vi "MaynuoM9714.vi"(4 "error in":T13, 7 "Command":T14) -> (0 "error out":T13, 3 "Response":T11)   [LabVIEW 2018]
uses:
  MOKO_LabViewLibrary/MokoLowLevel/MokoLowLovelControl/MLLC_Command.ctl
  MOKO_LabViewLibrary/MokoLowLevel/MokoLowLovelControl/MLLC_Error.ctl
  MOKO_LabViewLibrary/MokoLowLevel/MokoLowLovelControl/MLLC_Mode.ctl
  MOKO_LabViewLibrary/MokoLowLevel/MokoLowLovelControl/MLLC_Response.ctl
  MOKO_LabViewLibrary/MokoLowLevel/MokoLowLovelControl/MLLC_DriverName.ctl
  MOKO_LabViewLibrary/MokoLowLevel/MokoLowLovelControl/MLLC_Request.ctl
  MOKO_LabViewLibrary/MokoLowLevel/MokoLowLovelControl/MLLC_ErrorCode.ctl
  MOKO_LabViewLibrary/MokoLowLevel/MokoLowLovelControl/MLLC_ResponseInit.ctl
  MOKO_LabViewLibrary/MokoLowLevel/MokoLowLovelControl/MLLC_ConnectCluster.ctl
  MOKO_LabViewLibrary/MokoLowLevel/MokoLowLovelControl/MLLC_InterfaceType.ctl
  MOKO_LabViewLibrary/MokoLowLevel/MokoLowLovelControl/MLLC_OpenedSession.ctl
  MOKO_LabViewLibrary/MokoLowLevel/MokoLowLovelControl/MLLC_InterfaceSettings.ctl
  MOKO_LabViewLibrary/MokoLowLevel/MokoLowLovelControl/MLLC_InterfaceKind.ctl
  MOKO_LabViewLibrary/MokoLowLevel/MokoLowLovelControl/MLLC_Rs232Settings.ctl
  data/M97-98 Series DC Electronic Load LabVIEW Driver/M9700 Driver/86/vi.lib/M9700 Modbus.llb/CTL Register Address.ctl
  data/M97-98 Series DC Electronic Load LabVIEW Driver/M9700 Driver/86/vi.lib/M9700 Modbus.llb/CTL CMD Register.ctl
panel:
  in  "Settings":T6={"Saved Data"=variant, "Data"={"Connect"={"InterfaceType"=enum."VISA", "OpenedSession"="", "InterfaceSettings"={"Interface"=enum."GPIB", "EOS 4 read"=enum."LF (\\n)", "EOS 4 write"=enum."LF (\\n)", "TMO, ms"=5000, "Sett"=variant(cluster{"Baud Rate":u32, "Data Bits":u16, "Parity":u16, "Stop Bits":u16, "Flow Control":u16, "Eho":bool} {"Baud Rate"=75, "Data Bits"=0, "Parity"=0, "Stop Bits"=0, "Flow Control"=0, "Eho"=FALSE})}}}}
  in  "Response Init":T7
  in  "Error Code":T8=5475
  in  "Request":T9
  in  "Driver Name":T10="MaynuoM9714"
  in  "Mode":T12=enum."Check"
  # "MaynuoM9714"
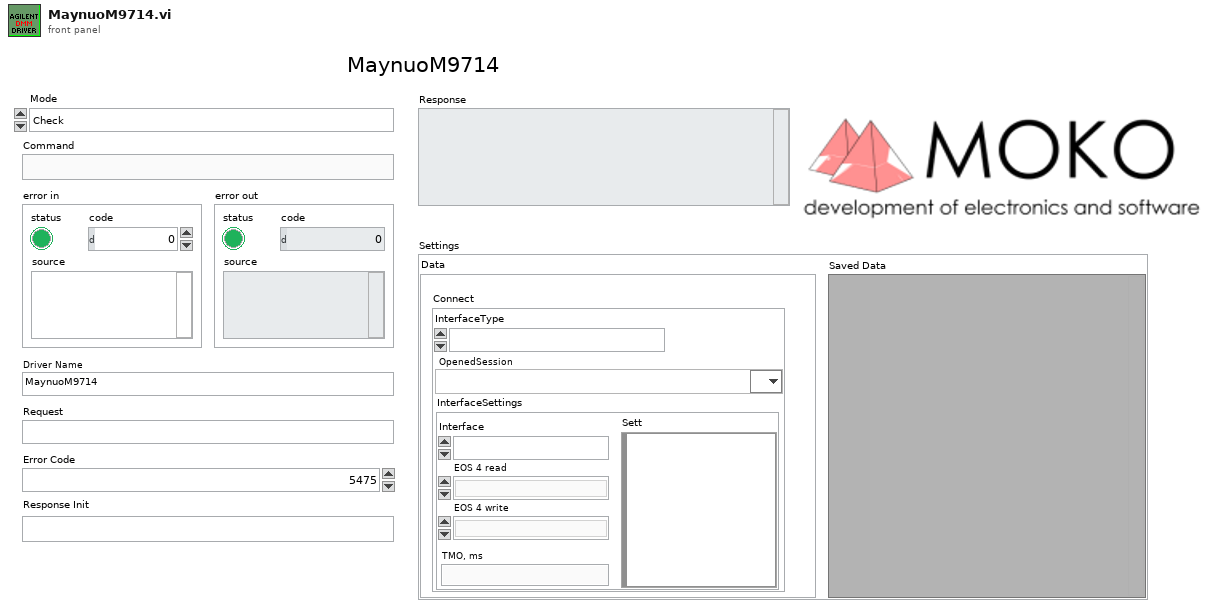
[diagram p1: front panel]
types:
  T1 = typedef "MLLC_ConnectCluster.ctl" = cluster{"InterfaceType":T2, "OpenedSession":T3, "InterfaceSettings":T4}
  T2 = typedef "MLLC_InterfaceType.ctl" = enum16{"VISA", "Prologix USB-GPIB"}
  T3 = typedef "MLLC_OpenedSession.ctl" = refnum<visa-resource-name>
  T4 = typedef "MLLC_InterfaceSettings.ctl" = cluster{"Interface":T5, "EOS 4 read":enum16{"Default (=EOS 4 write)", "CR (\\r)", "LF (\\n)", "None"}, "EOS 4 write":enum16{"CR+LF (\\r\\n)", "CR (\\r)", "LF (\\n)", "None"}, "TMO, ms":i32, "Sett":variant}
  T5 = typedef "MLLC_InterfaceKind.ctl" = enum16{"RS232", "GPIB", "USB", "Ethernet", "another"}
  T6 = cluster{"Saved Data":variant, "Data":cluster{"Connect":T1}}
  T7 = typedef "MLLC_ResponseInit.ctl" = string
  T8 = typedef "MLLC_ErrorCode.ctl" = u32
  T9 = typedef "MLLC_Request.ctl" = string
  T10 = typedef "MLLC_DriverName.ctl" = string
  T11 = typedef "MLLC_Response.ctl" = string
  T12 = typedef "MLLC_Mode.ctl" = enum16{"get", "set", "close", "Init", "Check"}
  T13 = typedef "MLLC_Error.ctl" = errorcluster
  T14 = typedef "MLLC_Command.ctl" = string
  T15 = typedef "MLLC_Rs232Settings.ctl" = cluster{"Baud Rate":u32, "Data Bits":u16, "Parity":u16, "Stop Bits":u16, "Flow Control":u16, "Eho":bool, "Address":dbl}
  T16 = typedef "CTL CMD Register.ctl" = u8
  T17 = typedef "CTL Register Address.ctl" = u16
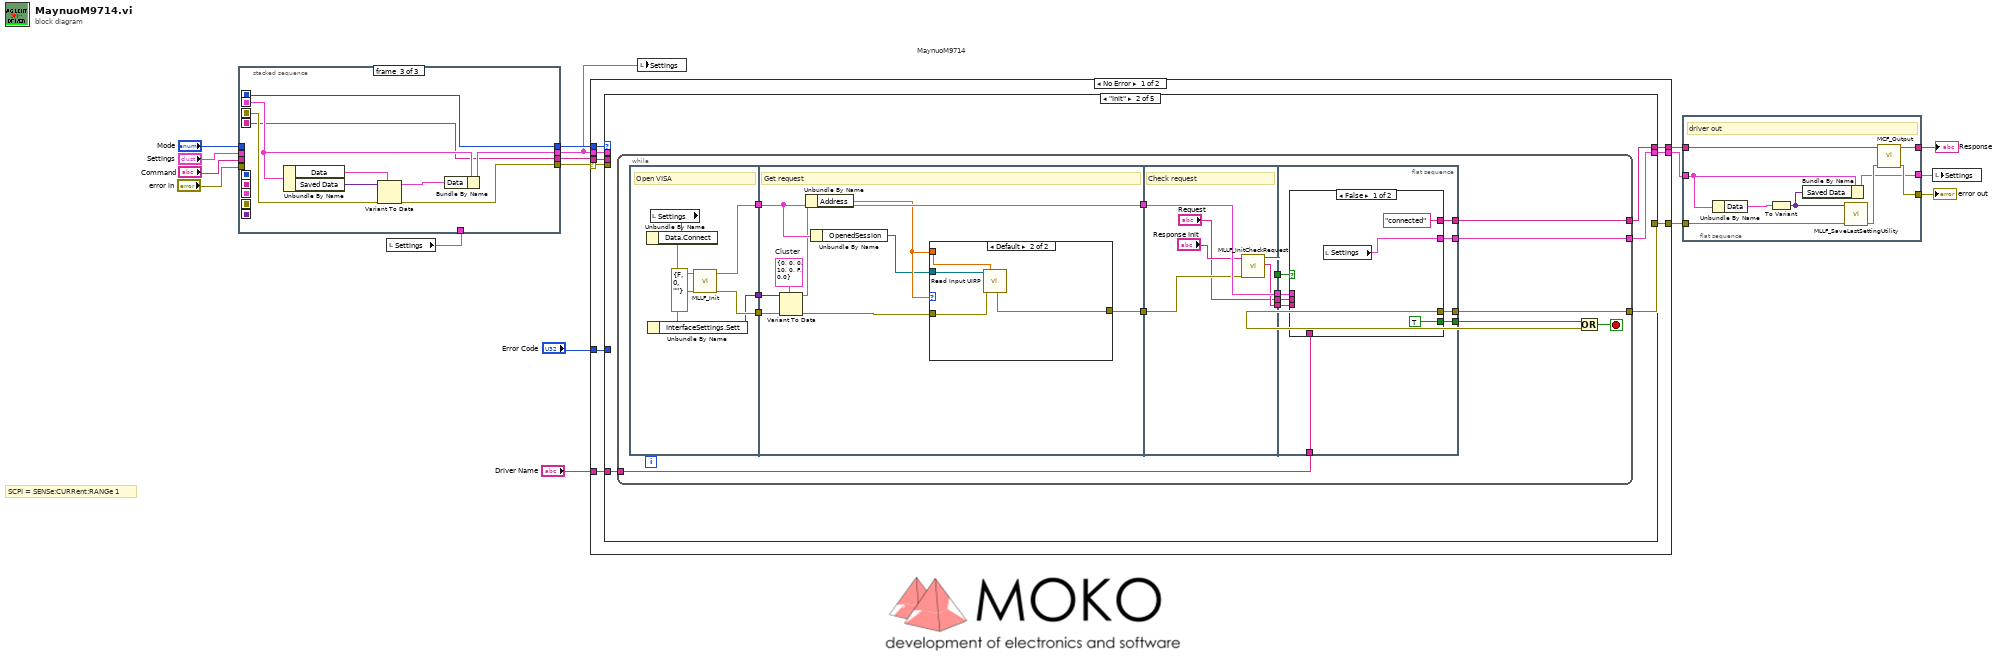
[diagram p0: block diagram]
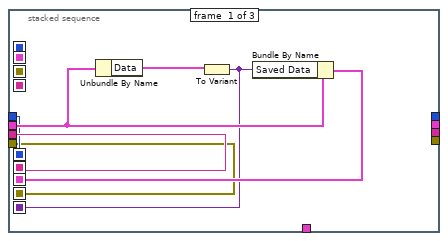
[diagram p2: hidden frame]
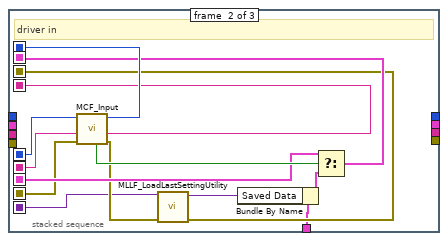
[diagram p3: hidden frame]
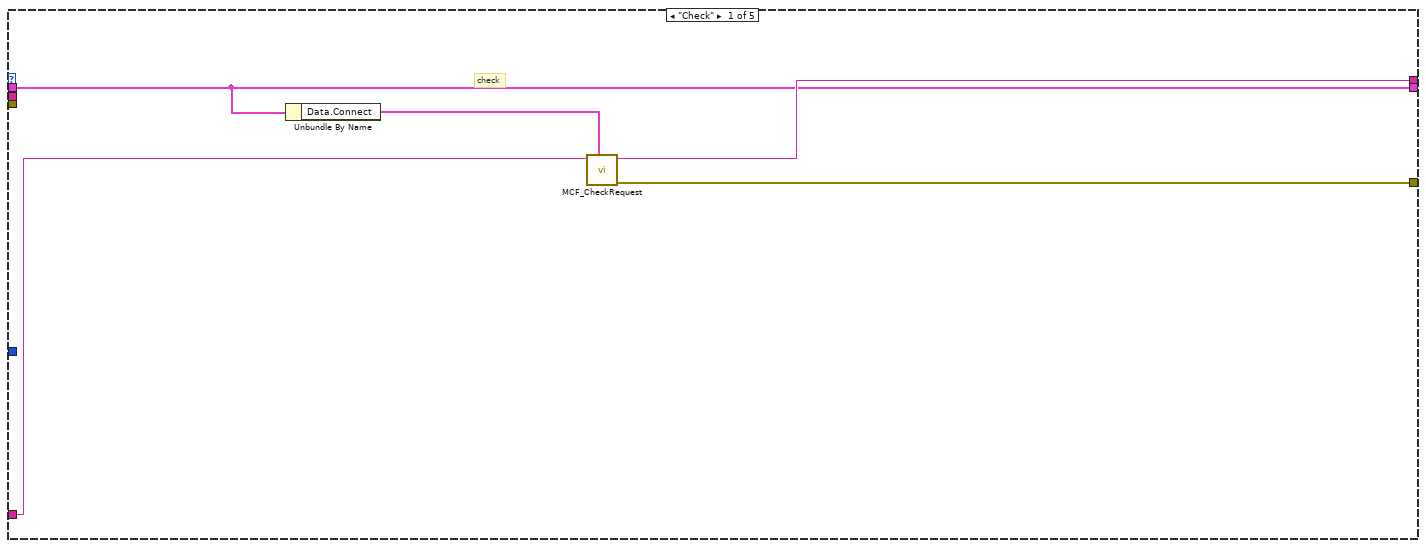
[diagram p4: hidden frame]
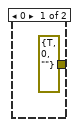
[diagram p5: hidden frame]
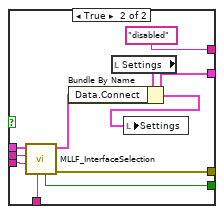
[diagram p6: hidden frame]
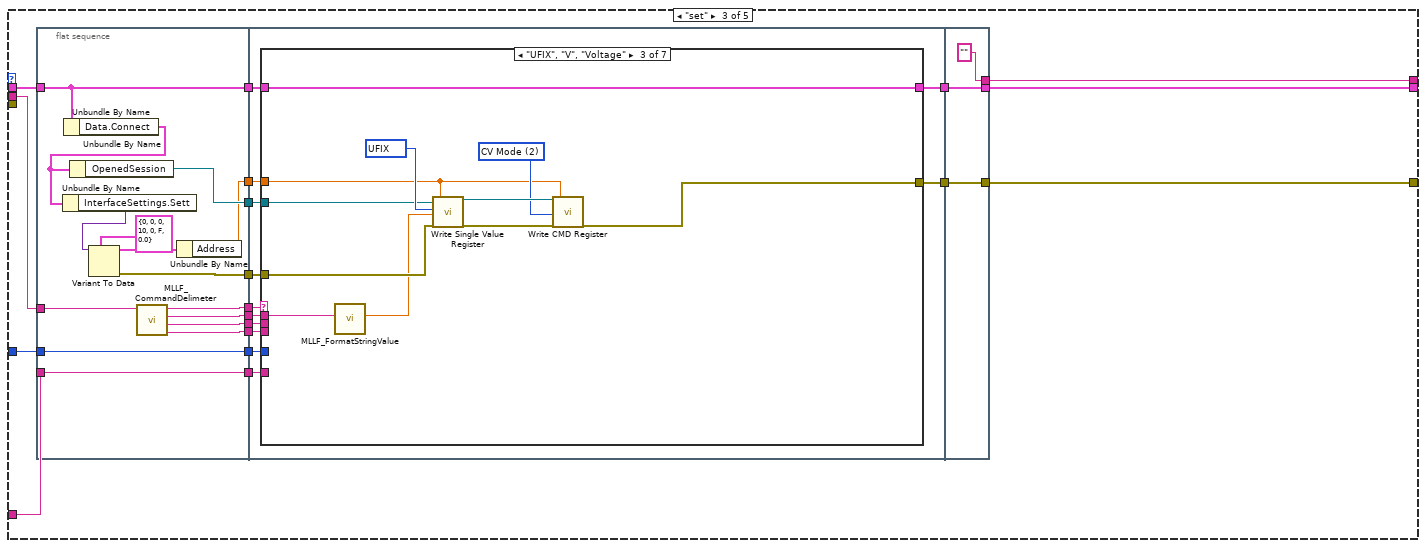
[diagram p7: hidden frame]
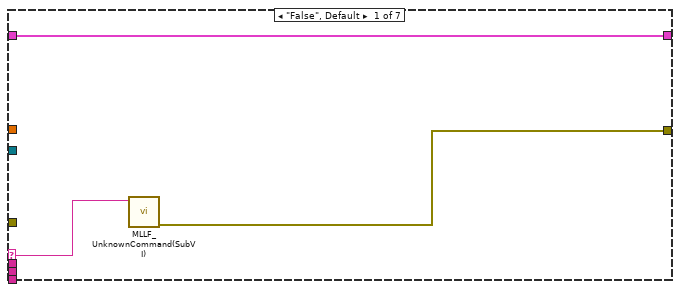
[diagram p8: hidden frame]
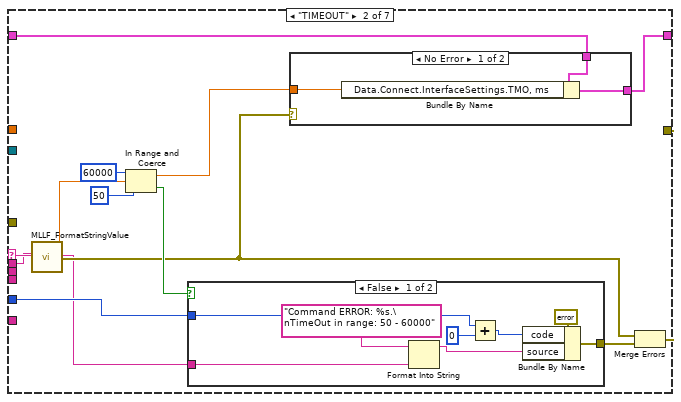
[diagram p9: hidden frame]
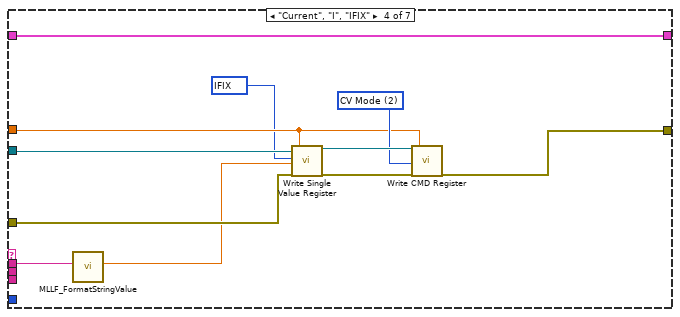
[diagram p12: hidden frame]
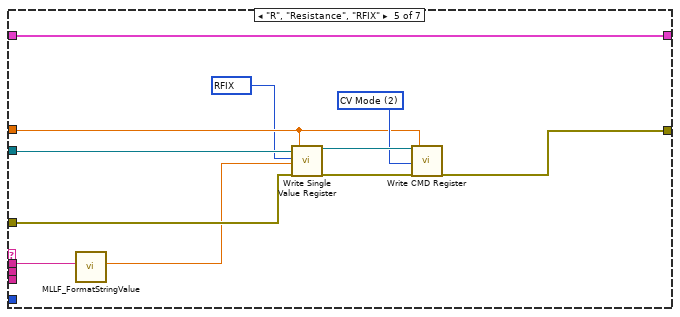
[diagram p13: hidden frame]
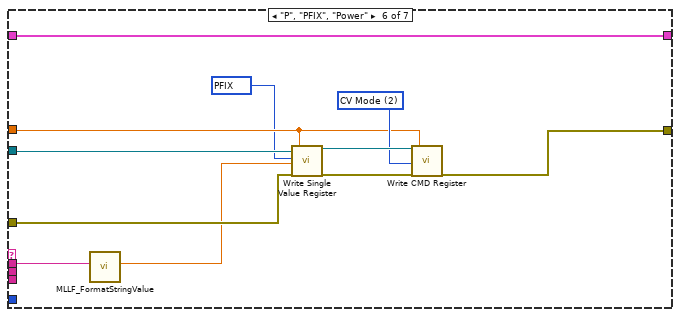
[diagram p14: hidden frame]
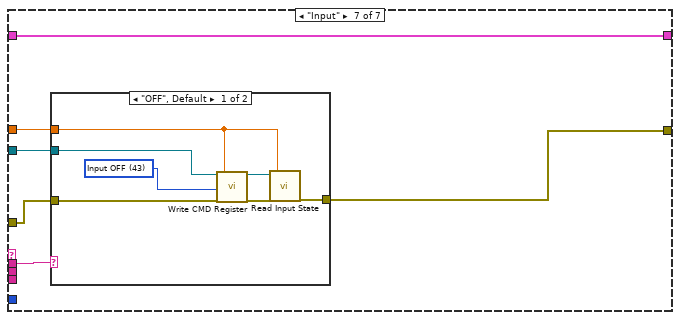
[diagram p15: hidden frame]
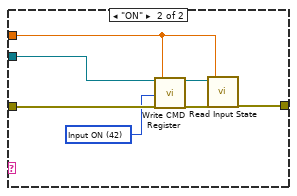
[diagram p16: hidden frame]
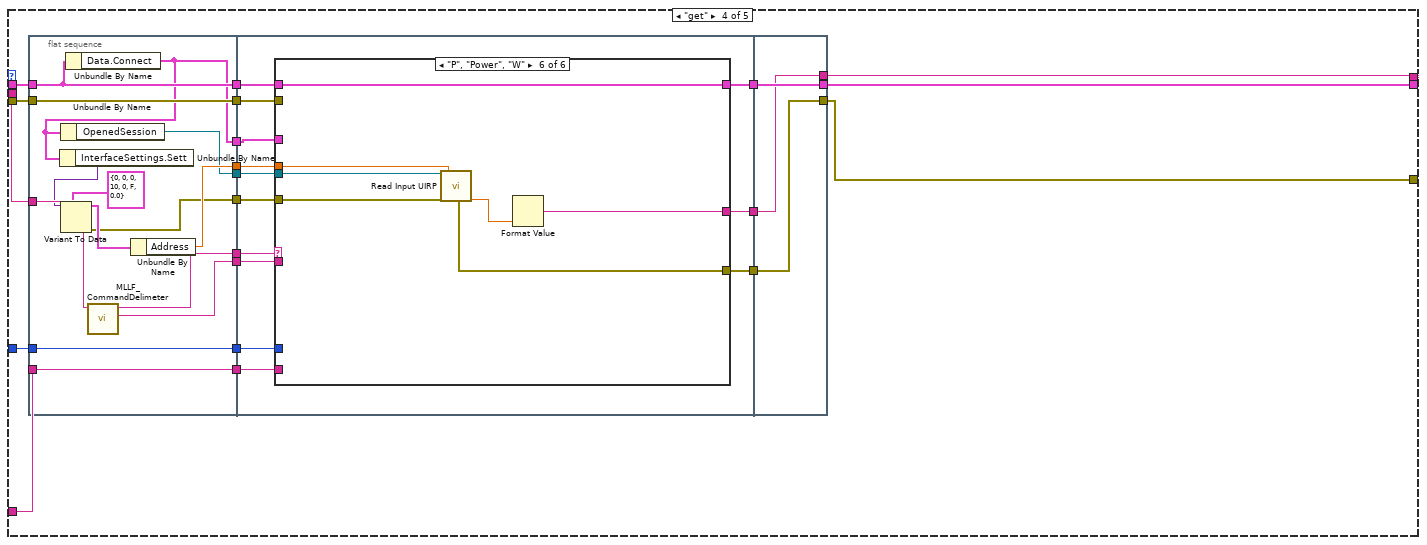
[diagram p17: hidden frame]
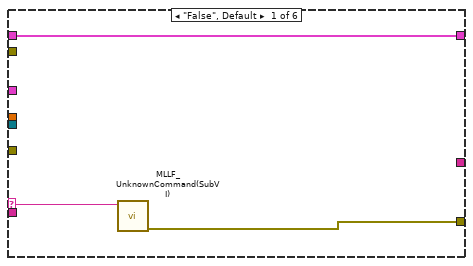
[diagram p18: hidden frame]
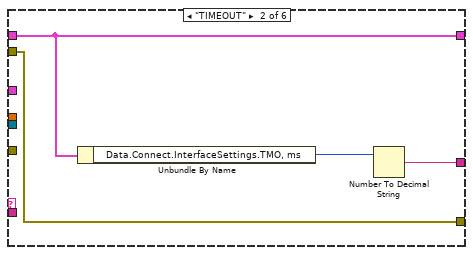
[diagram p19: hidden frame]
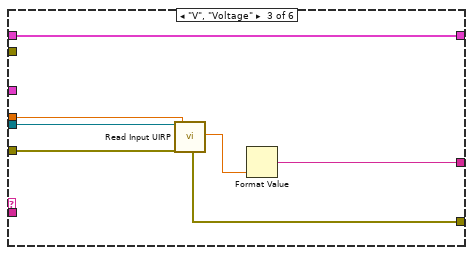
[diagram p20: hidden frame]
diagram:
  # "SCPI = SENSe:CURRent:RANGe 1"
  # "MaynuoM9714"
  n1 = local read "Settings"() -> (w8:T6)
  n2 = stacked-sequence {
    seq-local: [w20 _ _] -> [_ w36 _]
    seq-local: [w19 _ _] -> [_ w37 _]
    seq-local: [w22 _ _] -> [_ w32 _]
    seq-local: [w18 _ _] -> [_ w31 _]
    seq-local: [w21 _ _] -> [_ w27 _]
    seq-local: [_ w28 _] -> [_ _ w44]
    seq-local: [_ w38 _] -> [_ _ w41]
    seq-local: [_ w35 _] -> [_ _ w40]
    seq-local: [_ w34 _] -> [_ _ w45]
    tunnel: "Command" -> [w20 _ _]
    tunnel: "Mode" -> [w19 _ _]
    tunnel: "error in" -> [w18 _ _]
    tunnel: "Settings" -> [w23 _ _]
    tunnel: w8 -> [_ w26 _]
    tunnel: [_ _ w40] -> w10
    tunnel: [_ _ w43] -> w1
    tunnel: [_ _ w42] -> w9
    tunnel: [_ _ w41] -> w11
    frame #0 {
      n3 = Unbundle By Name(w23) -> ("Data"=w24:cluster{"Connect":T1})
      n4 = To Variant(anything=w24) -> (Variant=w21:variant)
      n5 = Bundle By Name(cluster=w23, "Saved Data"=w21) -> (w22:T6)
    }
    frame #1 {
      # "driver in"
      n6 = call "MCF_Input.vi"("Error In"=w31, "Command in"=w36, "Mode in"=w37) -> ("Error Out"=w30:errorcluster, "Command out"=w35:string, "Mode out"=w38:T12, "Boolean"=w33:bool)  [unwired: 5 in]
      n7 = call "MLLF_LoadLastSettingUtility.vi"("Error In"=w30, "Save data in"=w27) -> ("Error Out"=w28:errorcluster, "Save data out"=w25:variant)  [unwired: 8 in]
      n8 = Bundle By Name(cluster=w26, "Saved Data"=w25) -> (w29:T6)
      n9 = Select(t=w32, s=w33, f=w29) -> (s? t:f=w34:T6)
    }
    frame #2 {
      n10 = Unbundle By Name(w45) -> ("Data"=w46:cluster{"Connect":T1}, "Saved Data"=w39:variant)
      n11 = Variant To Data(error in=w44, type=w46, Variant=w39) -> (data=w47:cluster{"Connect":T1}, error out=w42:errorcluster)
      n12 = Bundle By Name(cluster=w45, "Data"=w47) -> (w43:T6)
    }
  }
  n13 = case shown="No Error" w9 {
    selector: w9 -> [w53 w362]
    tunnel: [w54 w362] -> w5
    tunnel: w11 -> [w56 _]
    tunnel: [w55 "An error occurred in the driver input module." ("String")] -> w7
    tunnel: w10 -> [w48 _]
    tunnel: w1 -> [w49 w361]
    tunnel: "Error Code" -> [w52 _]
    tunnel: "Driver Name" -> [w51 _]
    tunnel: [w50 w361] -> w6
    frame No Error {
      n14 = case shown="\"Init\"" w56 {
        tunnel: [w60 w65 w141 w273 "" ("String")] -> w55
        tunnel: [w61 w63 w144 w274 w358] -> w54
        tunnel: w53 -> [_ _ _ w287 _]
        tunnel: w52 -> [_ _ w147 w289 _]
        tunnel: w51 -> [w59 w62 w145 w288 _]
        tunnel: [w58 w64 w146 w290 w357] -> w50
        tunnel: w49 -> [w58 _ w133 w279 w357]
        tunnel: w48 -> [_ _ w132 w278 _]
        frame "Check" {
          # "check"
          n15 = Unbundle By Name(w58) -> ("Data.Connect"=w57:T1)
          n16 = call "MCF_CheckRequest.vi"("Permanent data.Connect"=w57, "Driver Name"=w59) -> ("Error Out"=w61:errorcluster, "Output String"=w60:string)  [unwired: 8 in]
        }
        frame "Init" {
          n17 = while {
            tunnel: [w71] -> w63
            tunnel: [w70] -> w65
            tunnel: [w69] -> w64
            tunnel: w62 -> [w73]
            stop <- w80 stop-if-true
            n18 = flat-sequence {
              tunnel: [w86] -> w79
              tunnel: [w85] -> w78
              tunnel: [w82] -> w66
              tunnel: w79 -> [w91]
              tunnel: w78 -> [w94]
              tunnel: [w95] -> w77
              tunnel: [w94] -> w76
              tunnel: w66 -> [w90]
              tunnel: w77 -> [w104]
              tunnel: w76 -> [w106]
              tunnel: [w106] -> w75
              tunnel: [w103] -> w74
              tunnel: [w102] -> w68
              tunnel: ["Request"] -> w67
              tunnel: w75 -> [w114]
              tunnel: w74 -> [w115]
              tunnel: w73 -> [w113]
              tunnel: [w112] -> w72
              tunnel: [w111] -> w71
              tunnel: [w110] -> w70
              tunnel: [w109] -> w69
              tunnel: w68 -> [w108]
              tunnel: w67 -> [w107]
              frame #0 {
                # "Open VISA"
                n19 = local read "Settings"() -> (w84:T6)
                n20 = Unbundle By Name(w84) -> ("Data.Connect"=w83:T1)
                n21 = Unbundle By Name(w83) -> ("InterfaceSettings.Sett"=w82:variant)
                n22 = call "MLLF_Init.vi"("Error In"=errorcluster {"status"=FALSE, "code"=0, "source"=""}, "DriverConnect in"=w83) -> ("Error Out"=w86:errorcluster, "DriverConnect out"=w85:T1)  [unwired: 6 in]
              }
              frame #1 {
                w92 = T15 {"Baud Rate"=0, "Data Bits"=0, "Parity"=0, "Stop Bits"=10, "Flow Control"=0, "Eho"=FALSE, "Address"=0.0}  # Cluster
                # "Get request"
                n23 = Variant To Data(error in=w91, type=w92, Variant=w90) -> (data=w93:T15, error out=w87:errorcluster)
                n24 = Unbundle By Name(w93) -> ("Address"=w89:dbl)
                n25 = Unbundle By Name(w94) -> ("OpenedSession"=w88:T3)
                n26 = case shown="Default" w89 {
                  tunnel: [errorcluster {"status"=TRUE, "code"=0, "source"=""} ("error out") w100] -> w95
                  tunnel: w88 -> [_ w99]
                  tunnel: w87 -> [_ w98]
                  tunnel: w89 -> [_ w97]
                  frame 0 {
                  }
                  frame Default {
                    n27 = call "Read Input UIRP.vi"("VISA resource name"=w99, "error in"=w98, "Load Address"=w97) -> ("error out"=w100:errorcluster)  [unwired: 16 out]
                  }
                }
              }
              frame #2 {
                # "Check request"
                n28 = call "MLLF_InitCheckRequest.vi"("error in (no error)"=w104, "Response Init"="Response Init") -> ("ResponseInit out"=w102:string, "Design"=w103:bool)  [unwired: 6 in, 2 out]
              }
              frame #3 {
                n29 = case shown="False" w115 {
                  tunnel: w114 -> [_ w127]
                  tunnel: [TRUE w122] -> w112
                  tunnel: [_ w125] -> w111
                  tunnel: ["connected" "disabled"] -> w110
                  tunnel: [w116 w123] -> w109
                  tunnel: w113 -> [_ w121]
                  tunnel: w108 -> [_ w120]
                  tunnel: w107 -> [_ w119]
                  frame False {
                    n30 = local read "Settings"() -> (w116:T6)
                  }
                  frame True {
                    n31 = call "MLLF_InterfaceSelection.vi"("Driver Name"=w121, "Response"=w120, "Request"=w119, "DriverConnect in"=w127) -> ("error out"=w125:T13, "DriverConnect out"=w126:T1, "stop init?"=w122:bool)  [unwired: 3 in, 2 out]
                    n32 = local read "Settings"() -> (w128:T6)
                    n33 = Bundle By Name(cluster=w128, "Data.Connect"=w126) -> (w123:T6)
                    n34 = local write "Settings"(w123) -> ()
                  }
                }
              }
            }
            n35 = Or(x=w72, y=w71) -> (x .or. y?=w80:bool)
          }
        }
        frame "set" {
          n36 = flat-sequence {
            tunnel: w145 -> [w161]
            tunnel: w133 -> [w155]
            tunnel: w147 -> [w162]
            tunnel: [w162] -> w140
            tunnel: [w155] -> w139
            tunnel: [w161] -> w138
            tunnel: [w156] -> w137
            tunnel: [w157] -> w136
            tunnel: [w158] -> w135
            tunnel: [w159] -> w134
            tunnel: w132 -> [w160]
            tunnel: [w152] -> w131
            tunnel: [w151] -> w130
            tunnel: [w150] -> w129
            tunnel: [w172] -> w143
            tunnel: [w168] -> w142
            tunnel: w140 -> [w174]
            tunnel: w139 -> [w173]
            tunnel: w138 -> [w171]
            tunnel: w137 -> [w170]
            tunnel: w136 -> [w169]
            tunnel: w135 -> [w167]
            tunnel: w134 -> [w166]
            tunnel: w131 -> [w165]
            tunnel: w130 -> [w164]
            tunnel: w129 -> [w163]
            tunnel: [w268] -> w144
            tunnel: [w269] -> w146
            tunnel: w143 -> [w269]
            tunnel: w142 -> [w268]
            tunnel: ["" ("String")] -> w141
            frame #0 {
              n37 = Unbundle By Name(w155) -> ("Data.Connect"=w149:T1)
              n38 = Unbundle By Name(w149) -> ("InterfaceSettings.Sett"=w148:variant)
              n39 = Unbundle By Name(w149) -> ("OpenedSession"=w152:T3)
              n40 = Variant To Data(type=T15 {"Baud Rate"=0, "Data Bits"=0, "Parity"=0, "Stop Bits"=10, "Flow Control"=0, "Eho"=FALSE, "Address"=0.0} ("Cluster"), Variant=w148) -> (data=w154:T15, error out=w150:errorcluster)  [unwired: 1 in]
              n41 = call "MLLF_CommandDelimeter.vi"("command with param"=w160) -> ("param 3"=w159:string, "param 2"=w158:string, "param 1"=w157:string, "command"=w156:string)  [unwired: 6 in, 1 out]
              n42 = Unbundle By Name(w154) -> ("Address"=w151:dbl)
            }
            frame #1 {
              n43 = case shown="\"UFIX\", \"V\", \"Voltage\"" w170 {
                selector: w170 -> [w176 w179 _ _ _ _ _]
                tunnel: w169 -> [_ w178 w204 w215 w226 w237 w247]
                tunnel: [w175 w184 w208 w220 w231 w242 w248] -> w168
                tunnel: w174 -> [_ w185 _ _ _ _ _]
                tunnel: w173 -> [w177 w189 w213 w224 w235 w246 w252]
                tunnel: [w177 w190 w213 w224 w235 w246 w252] -> w172
                tunnel: w171 -> [_ _ _ _ _ _ _]
                tunnel: w167 -> [_ _ _ _ _ _ _]
                tunnel: w166 -> [_ _ _ _ _ _ _]
                tunnel: w165 -> [_ _ w207 w219 w230 w241 w250]
                tunnel: w164 -> [_ _ w206 w218 w229 w240 w251]
                tunnel: w163 -> [_ _ w205 w217 w228 w239 w249]
                frame "False", Default {
                  n44 = call "MLLF_UnknownCommand(SubVI).vi"("Unknown command"=w176) -> ("error out"=w175:errorcluster)  [unwired: 10 in]
                }
                frame "TIMEOUT" {
                  n45 = call "MLLF_FormatStringValue.vi"("String Value"=w178) -> ("error out"=w180:T13, "number"=w181:dbl)  [unwired: 8 in, 1 out]
                  n46 = In Range and Coerce(upper limit=60000, x=w181, lower limit=50) -> (coerced(x)=w186:dbl, In Range?=w182:bool)
                  n47 = case shown="False" w182 {
                    tunnel: [w197 _] -> w183
                    tunnel: w185 -> [w196 _]
                    tunnel: w179 -> [w195 _]
                    frame False {
                      n48 = Format Into String(format string="Command ERROR: %s.\nTimeOut in range: 50 - 60000", w195) -> (resulting string=w199:string)  [unwired: 2 in, 1 out]
                      n49 = Add(x=w196, y=0) -> (x+y=w200:T8)
                      n50 = Bundle By Name(cluster=errorcluster {"status"=TRUE, "code"=0, "source"=""} ("error out"), "code"=w200, "source"=w199) -> (w197:errorcluster)
                    }
                    frame True {
                    }
                  }
                  n51 = case shown="No Error" w180 {
                    tunnel: [w193 w194] -> w190
                    tunnel: w189 -> [w192 w194]
                    tunnel: w186 -> [w191 _]
                    frame No Error {
                      n52 = Bundle By Name(cluster=w192, "Data.Connect.InterfaceSettings.TMO, ms"=w191) -> (w193:T6)
                    }
                    frame Error {
                    }
                  }
                  n53 = Merge Errors(w180, w183) -> (w184:errorcluster)
                }
                frame "UFIX", "V", "Voltage" {
                  w210 = T16 2 items=["CC Mode"=1, "CV Mode"=2, "CW Mode"=3, "CR Mode"=4, "Short Mode"=26, "Set SysPara"=41, "Input ON"=42, "Input OFF"=43] ("CMD Register Value")
                  w212 = T17 2563 items=["REMOTE"=1283, "ISTATE"=1296, "CMD"=2560, "IFIX"=2561, "UFIX"=2563, "PFIX"=2565, "RFIX"=2567, "IMAX"=2612, "UMAX"=2614, "PMAX"=2616, "U"=2816, "I"=2818, "MODEL"=2822, "EDITION"=2823] ("Register Address")
                  n54 = call "MLLF_FormatStringValue.vi"("String Value"=w204) -> ("number"=w203:dbl)  [unwired: 8 in, 2 out]
                  n55 = call "Write Single Value Register.vi"("VISA resource name"=w207, "Starting Address(HEX)"=w212, "Register Single Value"=w203, "error in"=w205, "Load Address"=w206) -> ("VISA resource name out"=w211:refnum<visa-resource-name>, "error out"=w209:errorcluster)  [unwired: 13 out]
                  n56 = call "Write CMD Register.vi"("VISA resource name"=w211, "CMD Value"=w210, "error in"=w209, "Load Address"=w206) -> ("error out"=w208:errorcluster)  [unwired: 15 out]
                }
                frame "Current", "I", "IFIX" {
                  w216 = T17 2561 items=["REMOTE"=1283, "ISTATE"=1296, "CMD"=2560, "IFIX"=2561, "UFIX"=2563, "PFIX"=2565, "RFIX"=2567, "IMAX"=2612, "UMAX"=2614, "PMAX"=2616, "U"=2816, "I"=2818, "MODEL"=2822, "EDITION"=2823] ("Register Address")
                  w222 = T16 2 items=["CC Mode"=1, "CV Mode"=2, "CW Mode"=3, "CR Mode"=4, "Short Mode"=26, "Set SysPara"=41, "Input ON"=42, "Input OFF"=43] ("CMD Register Value")
                  n57 = call "MLLF_FormatStringValue.vi"("String Value"=w215) -> ("number"=w214:dbl)  [unwired: 8 in, 2 out]
                  n58 = call "Write Single Value Register.vi"("VISA resource name"=w219, "Starting Address(HEX)"=w216, "Register Single Value"=w214, "error in"=w217, "Load Address"=w218) -> ("VISA resource name out"=w223:refnum<visa-resource-name>, "error out"=w221:errorcluster)  [unwired: 13 out]
                  n59 = call "Write CMD Register.vi"("VISA resource name"=w223, "CMD Value"=w222, "error in"=w221, "Load Address"=w218) -> ("error out"=w220:errorcluster)  [unwired: 15 out]
                }
                frame "R", "Resistance", "RFIX" {
                  w227 = T17 2567 items=["REMOTE"=1283, "ISTATE"=1296, "CMD"=2560, "IFIX"=2561, "UFIX"=2563, "PFIX"=2565, "RFIX"=2567, "IMAX"=2612, "UMAX"=2614, "PMAX"=2616, "U"=2816, "I"=2818, "MODEL"=2822, "EDITION"=2823] ("Register Address")
                  w233 = T16 2 items=["CC Mode"=1, "CV Mode"=2, "CW Mode"=3, "CR Mode"=4, "Short Mode"=26, "Set SysPara"=41, "Input ON"=42, "Input OFF"=43] ("CMD Register Value")
                  n60 = call "MLLF_FormatStringValue.vi"("String Value"=w226) -> ("number"=w225:dbl)  [unwired: 8 in, 2 out]
                  n61 = call "Write Single Value Register.vi"("VISA resource name"=w230, "Starting Address(HEX)"=w227, "Register Single Value"=w225, "error in"=w228, "Load Address"=w229) -> ("VISA resource name out"=w234:refnum<visa-resource-name>, "error out"=w232:errorcluster)  [unwired: 13 out]
                  n62 = call "Write CMD Register.vi"("VISA resource name"=w234, "CMD Value"=w233, "error in"=w232, "Load Address"=w229) -> ("error out"=w231:errorcluster)  [unwired: 15 out]
                }
                frame "P", "PFIX", "Power" {
                  w238 = T17 2565 items=["REMOTE"=1283, "ISTATE"=1296, "CMD"=2560, "IFIX"=2561, "UFIX"=2563, "PFIX"=2565, "RFIX"=2567, "IMAX"=2612, "UMAX"=2614, "PMAX"=2616, "U"=2816, "I"=2818, "MODEL"=2822, "EDITION"=2823] ("Register Address")
                  w244 = T16 2 items=["CC Mode"=1, "CV Mode"=2, "CW Mode"=3, "CR Mode"=4, "Short Mode"=26, "Set SysPara"=41, "Input ON"=42, "Input OFF"=43] ("CMD Register Value")
                  n63 = call "MLLF_FormatStringValue.vi"("String Value"=w237) -> ("number"=w236:dbl)  [unwired: 8 in, 2 out]
                  n64 = call "Write Single Value Register.vi"("VISA resource name"=w241, "Starting Address(HEX)"=w238, "Register Single Value"=w236, "error in"=w239, "Load Address"=w240) -> ("VISA resource name out"=w245:refnum<visa-resource-name>, "error out"=w243:errorcluster)  [unwired: 13 out]
                  n65 = call "Write CMD Register.vi"("VISA resource name"=w245, "CMD Value"=w244, "error in"=w243, "Load Address"=w240) -> ("error out"=w242:errorcluster)  [unwired: 15 out]
                }
                frame "Input" {
                  n66 = case shown="\"OFF\", Default" w247 {
                    tunnel: w251 -> [w257 w264]
                    tunnel: w250 -> [w254 w263]
                    tunnel: w249 -> [w256 w262]
                    tunnel: [w253 w261] -> w248
                    frame "OFF", Default {
                      w255 = T16 43 items=["CC Mode"=1, "CV Mode"=2, "CW Mode"=3, "CR Mode"=4, "Short Mode"=26, "Set SysPara"=41, "Input ON"=42, "Input OFF"=43] ("CMD Register Value")
                      n67 = call "Write CMD Register.vi"("VISA resource name"=w254, "CMD Value"=w255, "error in"=w256, "Load Address"=w257) -> ("VISA resource name out"=w259:refnum<visa-resource-name>, "error out"=w258:errorcluster)  [unwired: 14 out]
                      n68 = call "Read Input State.vi"("VISA resource name"=w259, "error in"=w258, "Load Address"=w257) -> ("error out"=w253:errorcluster)  [unwired: 16 out]
                    }
                    frame "ON" {
                      w260 = T16 42 items=["CC Mode"=1, "CV Mode"=2, "CW Mode"=3, "CR Mode"=4, "Short Mode"=26, "Set SysPara"=41, "Input ON"=42, "Input OFF"=43] ("CMD Register Value")
                      n69 = call "Write CMD Register.vi"("VISA resource name"=w263, "CMD Value"=w260, "error in"=w262, "Load Address"=w264) -> ("VISA resource name out"=w266:refnum<visa-resource-name>, "error out"=w265:errorcluster)  [unwired: 14 out]
                      n70 = call "Read Input State.vi"("VISA resource name"=w266, "error in"=w265, "Load Address"=w264) -> ("error out"=w261:errorcluster)  [unwired: 16 out]
                    }
                  }
                }
              }
            }
            frame #2 {
            }
          }
        }
        frame "get" {
          n71 = flat-sequence {
            tunnel: w287 -> [w302]
            tunnel: w288 -> [w303]
            tunnel: w289 -> [w304]
            tunnel: w279 -> [w298]
            tunnel: [w298] -> w286
            tunnel: [w304] -> w285
            tunnel: [w303] -> w284
            tunnel: [w293] -> w283
            tunnel: [w299] -> w282
            tunnel: [w300] -> w281
            tunnel: [w302] -> w280
            tunnel: w278 -> [w301]
            tunnel: [w294] -> w272
            tunnel: [w292] -> w271
            tunnel: [w291] -> w270
            tunnel: w286 -> [w317]
            tunnel: w285 -> [w315]
            tunnel: w284 -> [w314]
            tunnel: w283 -> [w312]
            tunnel: w282 -> [w311]
            tunnel: w281 -> [w310]
            tunnel: w280 -> [w308]
            tunnel: [w316] -> w277
            tunnel: [w313] -> w276
            tunnel: [w309] -> w275
            tunnel: w272 -> [w307]
            tunnel: w271 -> [w306]
            tunnel: w270 -> [w305]
            tunnel: [w355] -> w290
            tunnel: w277 -> [w355]
            tunnel: w276 -> [w353]
            tunnel: w275 -> [w354]
            tunnel: [w353] -> w274
            tunnel: [w354] -> w273
            frame #0 {
              n72 = Unbundle By Name(w298) -> ("Data.Connect"=w293:T1)
              n73 = Unbundle By Name(w293) -> ("InterfaceSettings.Sett"=w295:variant)
              n74 = Unbundle By Name(w293) -> ("OpenedSession"=w292:T3)
              n75 = Variant To Data(type=T15 {"Baud Rate"=0, "Data Bits"=0, "Parity"=0, "Stop Bits"=10, "Flow Control"=0, "Eho"=FALSE, "Address"=0.0} ("Cluster"), Variant=w295) -> (data=w297:T15, error out=w291:errorcluster)  [unwired: 1 in]
              n76 = call "MLLF_CommandDelimeter.vi"("command with param"=w301) -> ("param 1"=w300:string, "command"=w299:string)  [unwired: 6 in, 3 out]
              n77 = Unbundle By Name(w297) -> ("Address"=w294:dbl)
            }
            frame #1 {
              n78 = case shown="\"P\", \"Power\", \"W\"" w311 {
                selector: w311 -> [w319 _ _ _ _ _]
                tunnel: [w318 w323 w328 w336 w343 w350] -> w313
                tunnel: w315 -> [_ _ _ _ _ _]
                tunnel: [w320 w324 w331 w338 w345 w352] -> w316
                tunnel: w317 -> [w320 w324 w331 w338 w345 w352]
                tunnel: w312 -> [_ _ _ _ _ _]
                tunnel: w314 -> [_ _ _ _ _ _]
                tunnel: w310 -> [_ _ _ _ _ _]
                tunnel: [_ w321 w329 w337 w344 w351] -> w309
                tunnel: w308 -> [_ w323 _ _ _ _]
                tunnel: w307 -> [_ _ w327 w335 w342 w349]
                tunnel: w306 -> [_ _ w326 w334 w341 w348]
                tunnel: w305 -> [_ _ w325 w333 w340 w347]
                frame "False", Default {
                  n79 = call "MLLF_UnknownCommand(SubVI).vi"("Unknown command"=w319) -> ("error out"=w318:errorcluster)  [unwired: 10 in]
                }
                frame "TIMEOUT" {
                  n80 = Unbundle By Name(w324) -> ("Data.Connect.InterfaceSettings.TMO, ms"=w322:i32)
                  n81 = Number To Decimal String(number=w322) -> (decimal integer string=w321:string)  [unwired: 1 in]
                }
                frame "V", "Voltage" {
                  n82 = call "Read Input UIRP.vi"("VISA resource name"=w326, "error in"=w325, "Load Address"=w327) -> ("error out"=w328:errorcluster, "Actual Voltage(V)"=w330:sgl)  [unwired: 15 out]
                  n83 = Format Value(value (0)=w330) -> (output string=w329:string)  [unwired: 2 in]
                }
                frame "A", "Current", "I" {
                  n84 = call "Read Input UIRP.vi"("VISA resource name"=w334, "error in"=w333, "Load Address"=w335) -> ("error out"=w336:errorcluster, "Actual Current(A)"=w332:sgl)  [unwired: 15 out]
                  n85 = Format Value(value (0)=w332) -> (output string=w337:string)  [unwired: 2 in]
                }
                frame "Ohm", "R", "Resistance" {
                  n86 = call "Read Input UIRP.vi"("VISA resource name"=w341, "error in"=w340, "Load Address"=w342) -> ("error out"=w343:errorcluster, "Actual Resistance(Ohm)"=w339:sgl)  [unwired: 15 out]
                  n87 = Format Value(value (0)=w339) -> (output string=w344:string)  [unwired: 2 in]
                }
                frame "P", "Power", "W" {
                  n88 = call "Read Input UIRP.vi"("VISA resource name"=w348, "error in"=w347, "Load Address"=w349) -> ("error out"=w350:errorcluster, "Actual Power(W)"=w346:sgl)  [unwired: 15 out]
                  n89 = Format Value(value (0)=w346) -> (output string=w351:string)  [unwired: 2 in]
                }
              }
            }
            frame #2 {
            }
          }
        }
        frame "close" {
          n90 = Unbundle By Name(w357) -> ("Data.Connect.OpenedSession"=w359:T3)
          n91 = VISA Close(VISA resource name=w359) -> (error out=w358:errorcluster)  [unwired: 1 in]
        }
      }
    }
    frame Error {
    }
  }
  n92 = local write "Settings"(w1) -> ()
  n93 = flat-sequence {
    tunnel: [w371] -> w2
    tunnel: [w370] -> w4
    tunnel: w7 -> [w369]
    tunnel: w5 -> [w368]
    tunnel: w6 -> [w364]
    tunnel: [w366] -> w3
    frame #0 {
      # "driver out"
      n94 = Unbundle By Name(w364) -> ("Data"=w363:cluster{"Connect":T1})
      n95 = To Variant(anything=w363) -> (Variant=w365:variant)
      n96 = Bundle By Name(cluster=w364, "Saved Data"=w365) -> (w366:T6)
      n97 = call "MLLF_SaveLastSettingUtility.vi"("error in"=w368, "Saved Data"=w365) -> ("error out"=w367:T13)  [unwired: 8 in, 1 out]
      n98 = call "MCF_Output.vi"("Error In"=w367, "Input"=w369) -> ("Error Out"=w370:errorcluster, "Output"=w371:string)  [unwired: 8 in]
    }
  }
  n99 = local write "Settings"(w3) -> ()
  "error out" <- w4
  "Response" <- w2
